vi "测试报告摘要4.vi"(8 "打印?":bool, 10 "试验时间":timestamp) -> ()   [LabVIEW 2010]
uses:
  <vilib>/Utility/NIReport.llb/NI_report.lvclass
  全局量/试验配置信息.vi
  <vilib>/Utility/NIReport.llb/Append Report Text (str wrap).vi
  全局量/自动测试结果.vi
  <vilib>/addons/_office/word.llb/Word Easy Table (str).vi
  <vilib>/addons/_office/NI_ReportGenerationToolkit.lvlib
panel:
  in  "序号":i32
  out "XY图":cluster{"Y":dbl[], "Y":dbl[]}[](graph)
  # "T：打印\nF：保存"
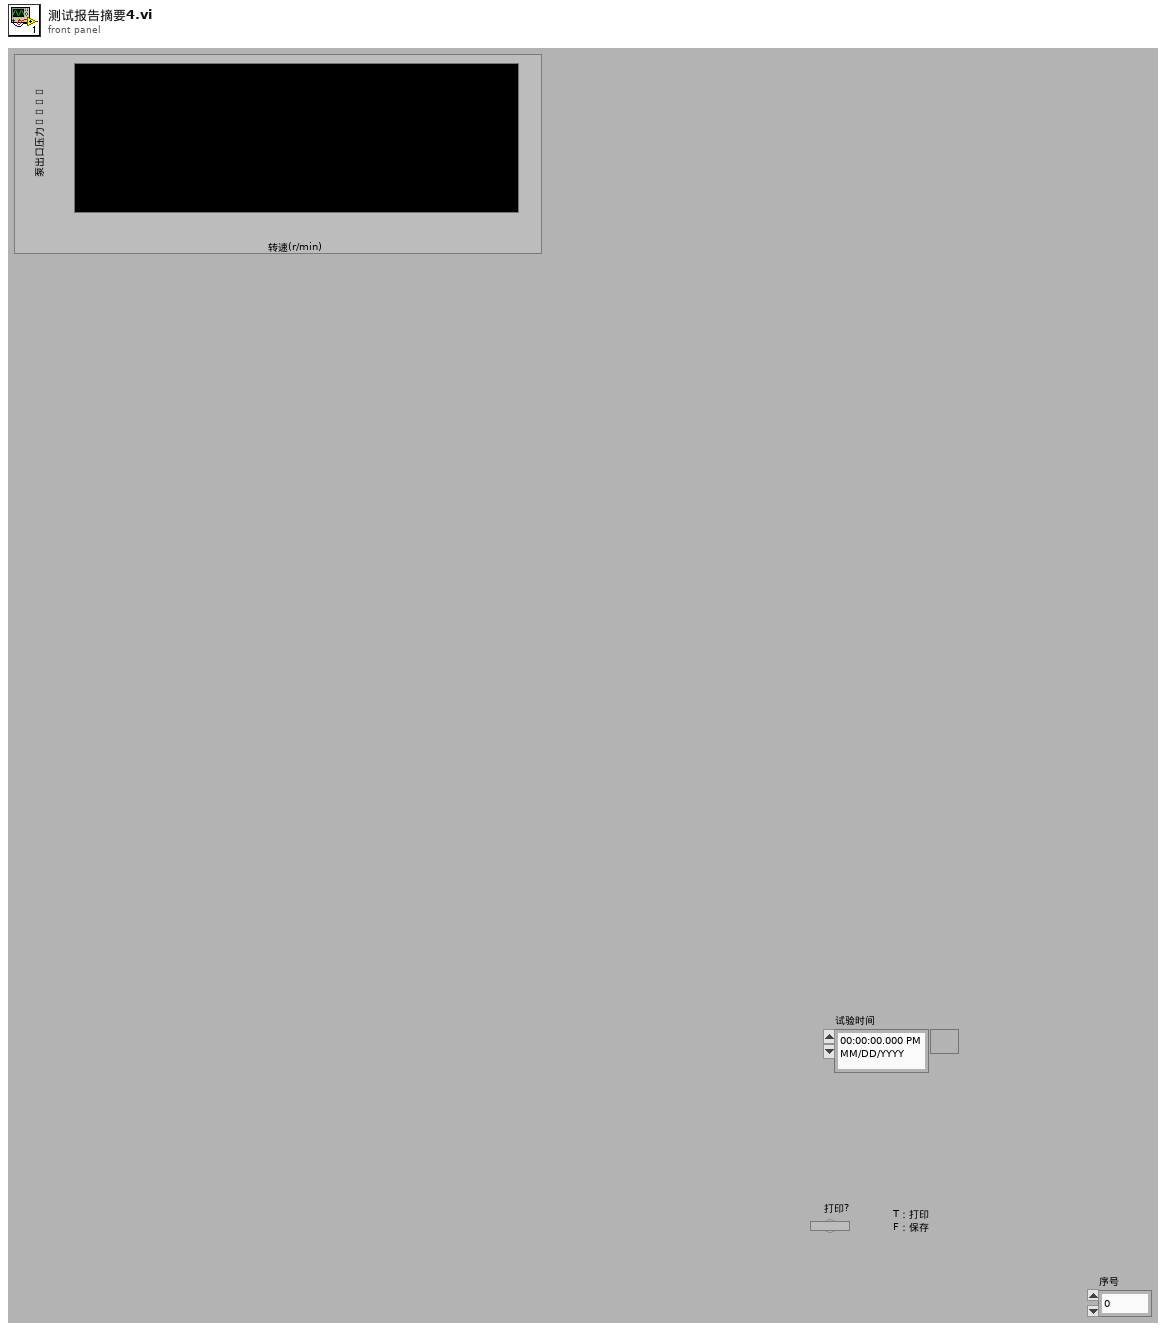
[diagram p1: front panel]
types:
  T1 = cluster{"position (Excel)":cluster{"row":i32, "column":i32}, "name (Excel)":string, "bookmark (Word)":string}
  T2 = enum16{"maximized", "minimized", "normal", "no change"}
  T3 = enum16{"Standard Report", "HTML", "Word", "Excel"}
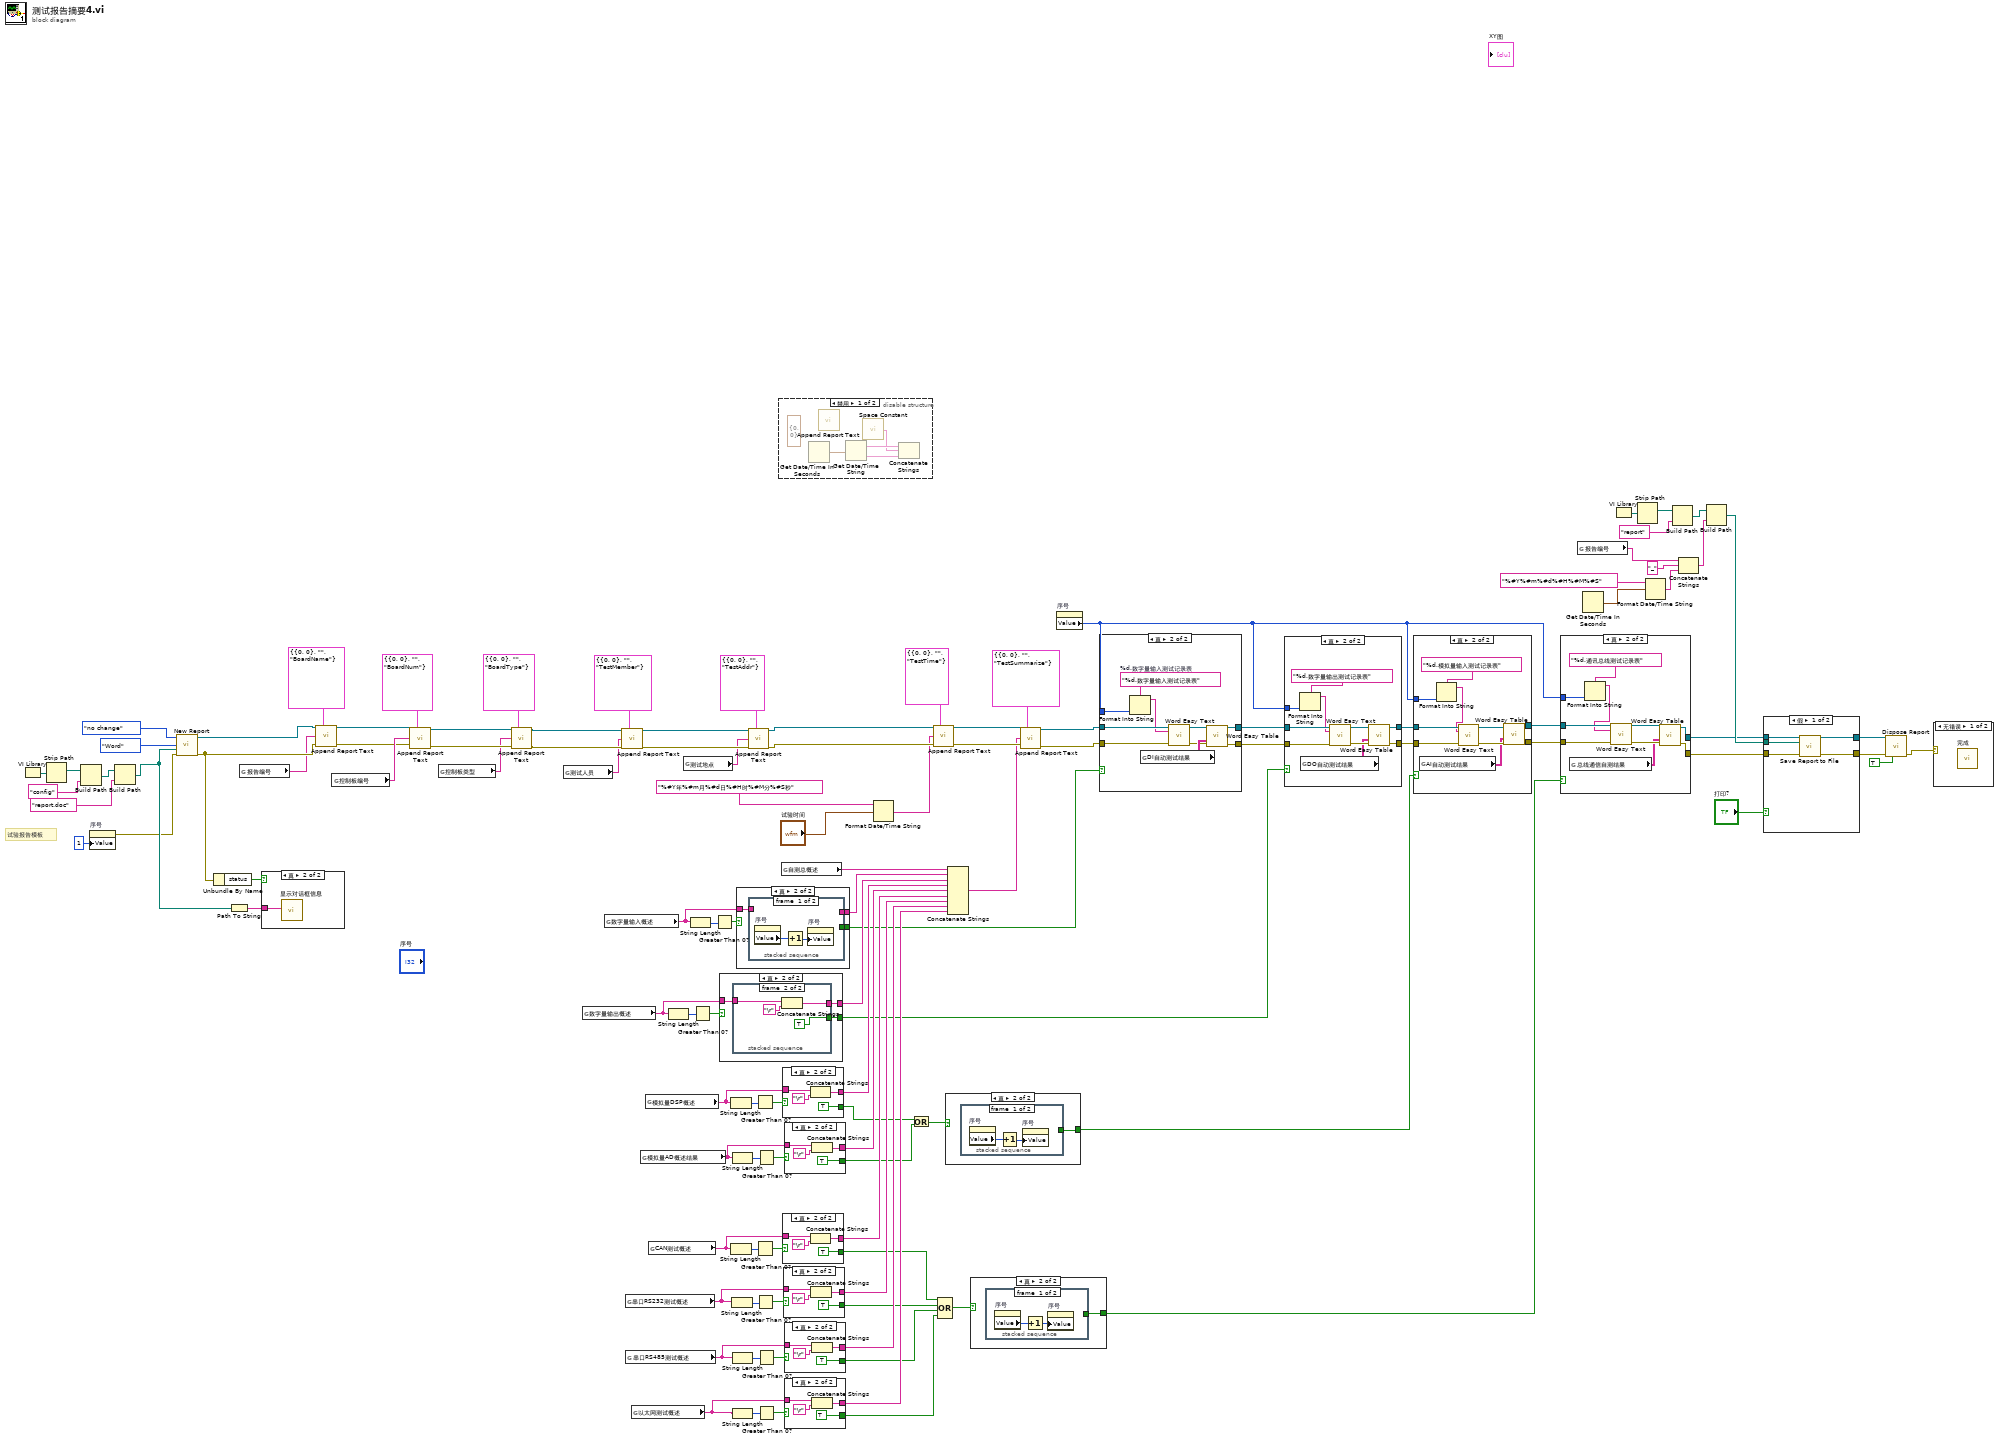
[diagram p0: block diagram]
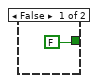
[diagram p2: hidden frame]
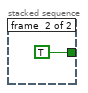
[diagram p3: hidden frame]
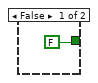
[diagram p4: hidden frame]
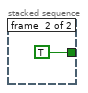
[diagram p5: hidden frame]
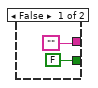
[diagram p10: hidden frame]
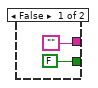
[diagram p11: hidden frame]
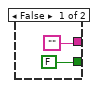
[diagram p12: hidden frame]
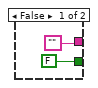
[diagram p13: hidden frame]
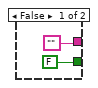
[diagram p14: hidden frame]
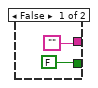
[diagram p15: hidden frame]
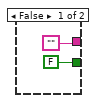
[diagram p16: hidden frame]
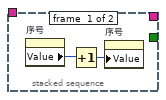
[diagram p17: hidden frame]
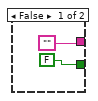
[diagram p18: hidden frame]
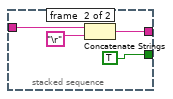
[diagram p19: hidden frame]
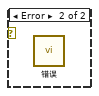
[diagram p20: hidden frame]
diagram:
  # "试验报告模板"
  n1 = VI Library() -> (path=w109:path)
  n2 = Strip Path(path=w109) -> (stripped path=w106:path)  [unwired: 1 out]
  n3 = Build Path(base path=w106, name or relative path="config") -> (appended path=w108:path)
  n4 = property on="序号" class="DigNum (严格)"("Value"=1 ("序号")) -> (error out=w18:errorcluster)  [unwired: 2 in, 1 out]
  n5 = Build Path(base path=w108, name or relative path="report.doc") -> (appended path=w112:path)
  n6 = call <vilib>:"New Report.vi"("window state (normal)"=T2."no change", "report type"=T3."Word", "template (empty)"=w112, "error in (no error)"=w18) -> ("report out"=w103:refnum<class "NI_report.lvclass">, "error out"=w102:errorcluster)  [unwired: 10 in]
  n7 = Unbundle By Name(w102) -> ("status"=w114:bool)
  n8 = Path To String(path=w112) -> (string=w113:string)
  n9 = global read "试验配置信息.vi" "报告编号"() -> (w71:string)
  n10 = case shown="真" w114 {
    tunnel: w113 -> [_ w115]
    frame False {
    }
    frame True {
      n11 = call "显示对话框信息"("Message"=w115) -> ()  [unwired: 9 in, 2 out]
    }
  }
  n12 = call-poly <vilib>:"Append Report Text.vi"("report in"=w103, "MS Office parameters"=T1 {"position (Excel)"={"row"=0, "column"=0}, "name (Excel)"="", "bookmark (Word)"="BoardName"}, "text"=w71, "error in (no error)"=w102) -> ("report out"=w85:refnum<class "NI_report.lvclass">, "error out"=w84:errorcluster)  [unwired: 8 in, 2 out]
  n13 = global read "试验配置信息.vi" "控制板编号"() -> (w86:string)
  n14 = call-poly <vilib>:"Append Report Text.vi"("report in"=w85, "MS Office parameters"=T1 {"position (Excel)"={"row"=0, "column"=0}, "name (Excel)"="", "bookmark (Word)"="BoardNum"}, "text"=w86, "error in (no error)"=w84) -> ("report out"=w98:refnum<class "NI_report.lvclass">, "error out"=w97:errorcluster)  [unwired: 8 in, 2 out]
  n15 = global read "试验配置信息.vi" "控制板类型"() -> (w83:string)
  n16 = call-poly <vilib>:"Append Report Text.vi"("report in"=w98, "MS Office parameters"=T1 {"position (Excel)"={"row"=0, "column"=0}, "name (Excel)"="", "bookmark (Word)"="BoardType"}, "text"=w83, "error in (no error)"=w97) -> ("report out"=w95:refnum<class "NI_report.lvclass">, "error out"=w94:errorcluster)  [unwired: 8 in, 2 out]
  n17 = global read "试验配置信息.vi" "测试人员"() -> (w88:string)
  n18 = global read "自动测试结果.vi" "数字量输出概述"() -> (w50:string)
  n19 = global read "自动测试结果.vi" "数字量输入概述"() -> (w51:string)
  n20 = call-poly <vilib>:"Append Report Text.vi"("report in"=w95, "MS Office parameters"=T1 {"position (Excel)"={"row"=0, "column"=0}, "name (Excel)"="", "bookmark (Word)"="TestMember"}, "text"=w88, "error in (no error)"=w94) -> ("report out"=w92:refnum<class "NI_report.lvclass">, "error out"=w91:errorcluster)  [unwired: 8 in, 2 out]
  n21 = global read "自动测试结果.vi" "串口RS232测试概述"() -> (w38:string)
  n22 = global read "自动测试结果.vi" "串口RS485测试概述"() -> (w33:string)
  n23 = global read "自动测试结果.vi" "以太网测试概述"() -> (w20:string)
  n24 = global read "自动测试结果.vi" "模拟量AD概述结果"() -> (w44:string)
  n25 = global read "自动测试结果.vi" "模拟量DSP概述"() -> (w45:string)
  n26 = global read "自动测试结果.vi" "CAN测试概述"() -> (w39:string)
  n27 = String Length(string=w50) -> (length=w48:i32)
  n28 = global read "试验配置信息.vi" "测试地点"() -> (w87:string)
  n29 = String Length(string=w51) -> (length=w53:i32)
  n30 = Greater Than 0?(x=w48) -> (x > 0?=w49:bool)
  n31 = Greater Than 0?(x=w53) -> (x > 0?=w52:bool)
  n32 = case shown="真" w49 {
    tunnel: w50 -> [_ w120]
    tunnel: ["" w119] -> w29
    tunnel: [FALSE w118] -> w16
    frame False {
    }
    frame True {
      n33 = stacked-sequence {
        tunnel: w120 -> [_ w126]
        tunnel: [_ w124] -> w119
        tunnel: [_ TRUE] -> w118
        frame #0 {
          n34 = property on="序号" class="DigNum (严格)"() -> ("Value"=w122:i32)  [unwired: 2 in, 2 out]
          n35 = Increment(x=w122) -> (x+1=w121:i32)
          n36 = property on="序号" class="DigNum (严格)"("Value"=w121) -> ()  [unwired: 2 in, 2 out]
        }
        frame #1 {
          n37 = Concatenate Strings(w126, "\r") -> (w124:string)
        }
      }
    }
  }
  n38 = String Length(string=w45) -> (length=w47:i32)
  n39 = String Length(string=w39) -> (length=w41:i32)
  n40 = String Length(string=w38) -> (length=w36:i32)
  n41 = String Length(string=w44) -> (length=w42:i32)
  n42 = String Length(string=w33) -> (length=w35:i32)
  n43 = String Length(string=w20) -> (length=w32:i32)
  n44 = case shown="真" w52 {
    tunnel: w51 -> [_ w131]
    tunnel: ["" w130] -> w30
    tunnel: [FALSE w129] -> w17
    frame False {
    }
    frame True {
      n45 = stacked-sequence {
        tunnel: w131 -> [_ w137]
        tunnel: [_ w135] -> w130
        tunnel: [_ TRUE] -> w129
        frame #0 {
          n46 = property on="序号" class="DigNum (严格)"() -> ("Value"=w132:i32)  [unwired: 2 in, 2 out]
          n47 = Increment(x=w132) -> (x+1=w133:i32)
          n48 = property on="序号" class="DigNum (严格)"("Value"=w133) -> ()  [unwired: 2 in, 2 out]
        }
        frame #1 {
          n49 = Concatenate Strings(w137, "\r") -> (w135:string)
        }
      }
    }
  }
  n50 = call-poly <vilib>:"Append Report Text.vi"("report in"=w92, "MS Office parameters"=T1 {"position (Excel)"={"row"=0, "column"=0}, "name (Excel)"="", "bookmark (Word)"="TestAddr"}, "text"=w87, "error in (no error)"=w91) -> ("report out"=w90:refnum<class "NI_report.lvclass">, "error out"=w89:errorcluster)  [unwired: 8 in, 2 out]
  n51 = Greater Than 0?(x=w47) -> (x > 0?=w46:bool)
  n52 = Greater Than 0?(x=w41) -> (x > 0?=w40:bool)
  n53 = Greater Than 0?(x=w36) -> (x > 0?=w37:bool)
  n54 = Greater Than 0?(x=w42) -> (x > 0?=w43:bool)
  n55 = Greater Than 0?(x=w35) -> (x > 0?=w34:bool)
  n56 = Greater Than 0?(x=w32) -> (x > 0?=w21:bool)
  n57 = disable-structure shown="禁用" {
    frame Disabled {
      (unwired) cluster{"row":i32, "column":i32} {"row"=0, "column"=0} ("position (excel)")
      n58 = Get Date/Time In Seconds() -> (seconds since 1Jan1904=w141:timestamp)
      n59 = call-poly <vilib>:"Append Report Text.vi"() -> ()  [unwired: 12 in, 4 out]
      n60 = Get Date/Time String(seconds (now)=w141) -> (date string=w140:string, time string=w139:string)  [unwired: 2 in]
      n61 = call <vilib>:"Space Constant.vi"() -> ("String"=w138:string)
      n62 = Concatenate Strings(w140, w138, w139) -> ()  [unwired: 1 out]
    }
    frame Enabled {
    }
  }
  n63 = global read "自动测试结果.vi" "自测总概述"() -> (w31:string)
  n64 = case shown="真" w46 {
    tunnel: w45 -> [_ w147]
    tunnel: ["" w145] -> w28
    tunnel: [FALSE TRUE] -> w15
    frame False {
    }
    frame True {
      n65 = Concatenate Strings(w147, "\r") -> (w145:string)
    }
  }
  n66 = case shown="真" w40 {
    tunnel: w39 -> [_ w153]
    tunnel: ["" w151] -> w26
    tunnel: [FALSE TRUE] -> w12
    frame False {
    }
    frame True {
      n67 = Concatenate Strings(w153, "\r") -> (w151:string)
    }
  }
  n68 = case shown="真" w37 {
    tunnel: w38 -> [_ w159]
    tunnel: ["" w157] -> w25
    tunnel: [FALSE TRUE] -> w11
    frame False {
    }
    frame True {
      n69 = Concatenate Strings(w159, "\r") -> (w157:string)
    }
  }
  n70 = case shown="真" w43 {
    tunnel: w44 -> [_ w165]
    tunnel: ["" w163] -> w27
    tunnel: [FALSE TRUE] -> w14
    frame False {
    }
    frame True {
      n71 = Concatenate Strings(w165, "\r") -> (w163:string)
    }
  }
  n72 = case shown="真" w34 {
    tunnel: w33 -> [_ w171]
    tunnel: ["" w169] -> w24
    tunnel: [FALSE TRUE] -> w10
    frame False {
    }
    frame True {
      n73 = Concatenate Strings(w171, "\r") -> (w169:string)
    }
  }
  n74 = case shown="真" w21 {
    tunnel: w20 -> [_ w177]
    tunnel: ["" w175] -> w23
    tunnel: [FALSE TRUE] -> w9
    frame False {
    }
    frame True {
      n75 = Concatenate Strings(w177, "\r") -> (w175:string)
    }
  }
  n76 = Format Date/Time String(time format string (%c)="%#Y年%#m月%#d日%#H时%#M分%#S秒" ("时间格式字符串(%c)"), seconds (now)="试验时间") -> (date/time string=w60:string)  [unwired: 1 in]
  n77 = Or(x=w15, y=w14) -> (x .or. y?=w13:bool)
  n78 = call-poly <vilib>:"Append Report Text.vi"("report in"=w90, "MS Office parameters"=T1 {"position (Excel)"={"row"=0, "column"=0}, "name (Excel)"="", "bookmark (Word)"="TestTime"}, "text"=w60, "error in (no error)"=w89) -> ("report out"=w57:refnum<class "NI_report.lvclass">, "error out"=w56:errorcluster)  [unwired: 8 in, 2 out]
  n79 = Compound Arithmetic op=OR(w12, w11, w10, w9) -> (w8:bool)
  n80 = case shown="真" w13 {
    tunnel: [FALSE w179] -> w7
    frame False {
    }
    frame True {
      n81 = stacked-sequence {
        tunnel: [_ TRUE] -> w179
        frame #0 {
          n82 = property on="序号" class="DigNum (严格)"() -> ("Value"=w181:i32)  [unwired: 2 in, 2 out]
          n83 = Increment(x=w181) -> (x+1=w180:i32)
          n84 = property on="序号" class="DigNum (严格)"("Value"=w180) -> ()  [unwired: 2 in, 2 out]
        }
        frame #1 {
        }
      }
    }
  }
  n85 = Concatenate Strings(w31, w30, w29, w28, w27, w26, w25, w24, w23) -> (w22:string)
  n86 = case shown="真" w8 {
    tunnel: [FALSE w184] -> w5
    frame False {
    }
    frame True {
      n87 = stacked-sequence {
        tunnel: [_ TRUE] -> w184
        frame #0 {
          n88 = property on="序号" class="DigNum (严格)"() -> ("Value"=w186:i32)  [unwired: 2 in, 2 out]
          n89 = Increment(x=w186) -> (x+1=w185:i32)
          n90 = property on="序号" class="DigNum (严格)"("Value"=w185) -> ()  [unwired: 2 in, 2 out]
        }
        frame #1 {
        }
      }
    }
  }
  n91 = call-poly <vilib>:"Append Report Text.vi"("report in"=w57, "MS Office parameters"=T1 {"position (Excel)"={"row"=0, "column"=0}, "name (Excel)"="", "bookmark (Word)"="TestSummarize"}, "text"=w22, "error in (no error)"=w56) -> ("report out"=w55:refnum<class "NI_report.lvclass">, "error out"=w54:errorcluster)  [unwired: 8 in, 2 out]
  n92 = property on="序号" class="DigNum (严格)"() -> ("Value"=w6:i32)  [unwired: 2 in, 2 out]
  n93 = case shown="真" w17 {
    tunnel: [w189 w197] -> w67
    tunnel: [w188 w196] -> w65
    tunnel: w55 -> [w189 w194]
    tunnel: w54 -> [w188 w193]
    tunnel: w6 -> [_ w190]
    frame False {
    }
    frame True {
      w192 = "%d.数字量输入测试记录表"  # %d.数字量输入测试记录表
      n94 = Format Into String(format string=w192, w190) -> (resulting string=w191:string)  [unwired: 2 in, 1 out]
      n95 = global read "自动测试结果.vi" "DI自动测试结果"() -> (w199:string[][])
      n96 = call <vilib>:"Word Easy Text.vi"("report in"=w194, "text"=w191, "error in (no error)"=w193) -> ("report out"=w198:refnum<class "NI_report.lvclass">, "error out"=w195:errorcluster)  [unwired: 10 in, 1 out]
      n97 = call-poly <vilib>:"Word Easy Table.vi"("report in"=w198, "data"=w199, "error in (no error)"=w195) -> ("report out"=w197:refnum<class "NI_report.lvclass">, "error out"=w196:errorcluster)  [unwired: 10 in, 1 out]
    }
  }
  n98 = case shown="真" w16 {
    tunnel: w67 -> [w201 w211]
    tunnel: [w201 w209] -> w66
    tunnel: w65 -> [w200 w208]
    tunnel: [w200 w206] -> w64
    tunnel: w6 -> [_ w203]
    frame False {
    }
    frame True {
      n99 = Format Into String(format string="%d.数字量输出测试记录表", w203) -> (resulting string=w202:string)  [unwired: 2 in, 1 out]
      n100 = global read "自动测试结果.vi" "DO自动测试结果"() -> (w205:string[][])
      n101 = call <vilib>:"Word Easy Text.vi"("report in"=w211, "text"=w202, "error in (no error)"=w208) -> ("report out"=w210:refnum<class "NI_report.lvclass">, "error out"=w207:errorcluster)  [unwired: 10 in, 1 out]
      n102 = call-poly <vilib>:"Word Easy Table.vi"("report in"=w210, "data"=w205, "error in (no error)"=w207) -> ("report out"=w209:refnum<class "NI_report.lvclass">, "error out"=w206:errorcluster)  [unwired: 10 in, 1 out]
    }
  }
  n103 = case shown="真" w7 {
    tunnel: w66 -> [w213 w223]
    tunnel: w64 -> [w212 w221]
    tunnel: [w213 w219] -> w63
    tunnel: [w212 w218] -> w62
    tunnel: w6 -> [_ w215]
    frame False {
    }
    frame True {
      n104 = global read "自动测试结果.vi" "AI自动测试结果"() -> (w217:string[][])
      n105 = Format Into String(format string="%d.模拟量输入测试记录表", w215) -> (resulting string=w214:string)  [unwired: 2 in, 1 out]
      n106 = call <vilib>:"Word Easy Text.vi"("report in"=w223, "text"=w214, "error in (no error)"=w221) -> ("report out"=w222:refnum<class "NI_report.lvclass">, "error out"=w220:errorcluster)  [unwired: 10 in, 1 out]
      n107 = call-poly <vilib>:"Word Easy Table.vi"("report in"=w222, "data"=w217, "error in (no error)"=w220) -> ("report out"=w219:refnum<class "NI_report.lvclass">, "error out"=w218:errorcluster)  [unwired: 10 in, 1 out]
    }
  }
  n108 = case shown="真" w5 {
    tunnel: [w225 w235] -> w69
    tunnel: [w224 w234] -> w68
    tunnel: w63 -> [w225 w233]
    tunnel: w62 -> [w224 w232]
    tunnel: w6 -> [_ w227]
    frame False {
    }
    frame True {
      n109 = global read "自动测试结果.vi" "总线通信自测结果"() -> (w229:string[][])
      n110 = Format Into String(format string="%d.通讯总线测试记录表", w227) -> (resulting string=w226:string)  [unwired: 2 in, 1 out]
      n111 = call <vilib>:"Word Easy Text.vi"("report in"=w233, "text"=w226, "error in (no error)"=w232) -> ("report out"=w231:refnum<class "NI_report.lvclass">, "error out"=w230:errorcluster)  [unwired: 10 in, 1 out]
      n112 = call-poly <vilib>:"Word Easy Table.vi"("report in"=w231, "data"=w229, "error in (no error)"=w230) -> ("report out"=w235:refnum<class "NI_report.lvclass">, "error out"=w234:errorcluster)  [unwired: 10 in, 1 out]
    }
  }
  n113 = global read "试验配置信息.vi" "报告编号"() -> (w3:string)
  n114 = Get Date/Time In Seconds() -> (seconds since 1Jan1904=w77:timestamp)
  n115 = VI Library() -> (path=w78:path)
  n116 = Strip Path(path=w78) -> (stripped path=w81:path)  [unwired: 1 out]
  n117 = Format Date/Time String(time format string (%c)="%#Y%#m%#d%#H%#M%#S" ("时间格式字符串(%c)"), seconds (now)=w77) -> (date/time string=w4:string)  [unwired: 1 in]
  n118 = Build Path(base path=w81, name or relative path="report") -> (appended path=w79:path)
  n119 = Concatenate Strings(w3, "_", w4) -> (w1:string)
  n120 = Build Path(base path=w79, name or relative path=w1) -> (appended path=w72:path)
  n121 = case shown="假" "打印?" {
    tunnel: w69 -> [w240 w244]
    tunnel: w68 -> [w239 w243]
    tunnel: [w238 w242] -> w75
    tunnel: [w237 w241] -> w74
    tunnel: w72 -> [w236 _]
    frame False {
      n122 = call-dynamic "Save Report to File.vi"("report in"=w240, "report file path"=w236, "error in (no error)"=w239) -> ("report out"=w238:refnum<class "NI_report.lvclass">, "error out"=w237:errorcluster)  [unwired: 11 in]
    }
    frame True {
      n123 = call-dynamic "Print Report.vi"("report in"=w244, "error in (no error)"=w243) -> ("report out"=w242:refnum<class "NI_report.lvclass">, "error out"=w241:errorcluster)  [unwired: 12 in]
    }
  }
  n124 = call-dynamic "Dispose Report.vi"("report in"=w75, "error in (no error)"=w74, "close report? (T)"=TRUE) -> ("error out"=w70:errorcluster)  [unwired: 12 in]
  n125 = case shown="无错误" w70 {
    frame No Error {
      n126 = call "完成"() -> ()  [unwired: 10 in, 2 out]
    }
    frame Error {
      n127 = call "错误"() -> ()  [unwired: 10 in, 2 out]
    }
  }
